vi "niRFSTS RFPM Close.vi"(11 "TSM Context":T1) -> (0 "error out":errorcluster)   [LabVIEW 2014]
uses:
  <vilib>/NI_TestStand_SemiconductorModule/NI_TestStand_Semiconductor_Module.lvlibp/PinMap/General/SemiconductorModuleContext.ctl
  <vilib>/FPGAPlugInAG/Dynamic/niLvFpga_Close_Dynamic.vi
  <vilib>/rvi/interface/nirviCloseFPGA/nirviCloseFPGA.xnode
  <vilib>/NI_TestStand_SemiconductorModule/NI_TestStand_Semiconductor_Module.lvlibp
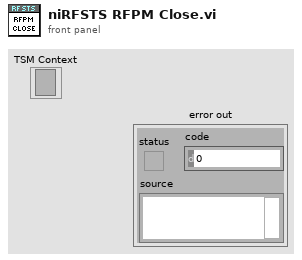
[diagram p1: front panel]
types:
  T1 = typedef "NI_TestStand_Semiconductor_Module.lvlibp/SemiconductorModuleContext.ctl" = refnum<k7>
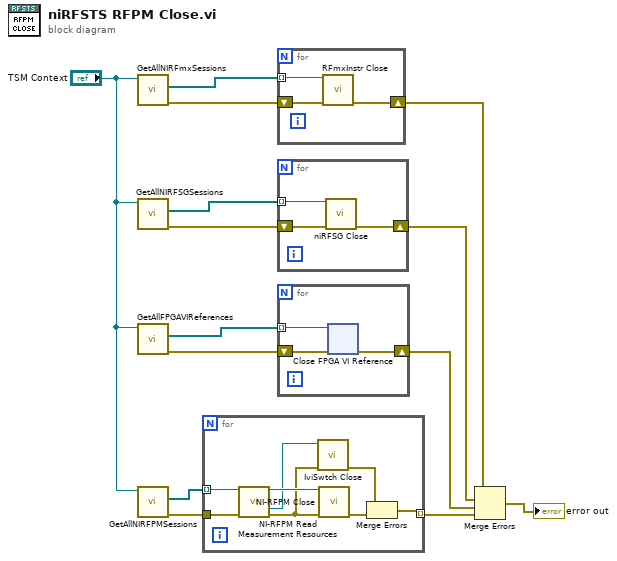
[diagram p0: block diagram]
diagram:
  n1 = call <vilib>:"GetAllNIRFmxSessions.vi"("Semiconductor Module Context"="TSM Context") -> ("error out"=w11:errorcluster, "Instrument Sessions"=w12:refnum<k21>[])  [unwired: 8 in, 1 out]
  n2 = call <vilib>:"GetAllNIRFSGSessions.vi"("Semiconductor Module Context"="TSM Context") -> ("error out"=w10:errorcluster, "Instrument Sessions"=w9:refnum<k15>[])  [unwired: 8 in, 1 out]
  n3 = call <vilib>:"GetAllFPGAVIReferences.vi"("Semiconductor Module Context"="TSM Context") -> ("error out"=w8:errorcluster, "FPGA VI References"=w7:refnum<k20>[])  [unwired: 8 in, 1 out]
  n4 = call <vilib>:"GetAllNIRFPMSessions.vi"("Semiconductor Module Context"="TSM Context") -> ("error out"=w1:errorcluster, "Instrument Sessions"=w2:refnum<k15>[])  [unwired: 8 in, 1 out]
  n5 = for {
    tunnel: w2 -> [w20] mode=indexing
    tunnel: w1 -> [w19]
    tunnel: [w22] -> w14 mode=indexing
    n6 = call <instrlib>:"NI-RFPM Read Measurement Resources.vi"("NI-5530 handle in"=w20, "error in"=w19) -> ("NI-5530 handle out"=w18:refnum<k15>, "Switch handle"=w16:refnum<k15>, "error out"=w17:errorcluster)  [unwired: 9 in, 2 out]
    n7 = call <vilib>:"IviSwtch Close.vi"("error in (no error)"=w17, "instrument handle"=w16) -> ("error out"=w15:errorcluster)  [unwired: 9 in]
    n8 = call <instrlib>:"NI-RFPM Close.vi"("NI-5530 handle in"=w18, "error in"=w17) -> ("error out"=w21:errorcluster)  [unwired: 13 in]
    n9 = Merge Errors(w15, w21) -> (w22:errorcluster)
  }
  n10 = for {
    tunnel: w12 -> [w25] mode=indexing
    shift-right: [w23] -> w6
    shift-left: w11 -> [w24]
    n11 = call <vilib>:"RFmxInstr Close.vi"("Instrument Handle In"=w25, "error in (no error)"=w24) -> ("error out"=w23:errorcluster)  [unwired: 13 in]
  }
  n12 = for {
    shift-right: [w27] -> w5
    shift-left: w10 -> [w28]
    tunnel: w9 -> [w26] mode=indexing
    n13 = call <instrlib>:"niRFSG Close.vi"("instrument handle"=w26, "error in"=w28) -> ("error out"=w27:errorcluster)  [unwired: 13 in]
  }
  n14 = for {
    shift-right: [w30] -> w4
    shift-left: w8 -> [w31]
    tunnel: w7 -> [w29] mode=indexing
    n15 = xnode "Close FPGA VI Reference"("FPGA VI Reference In"=w29, "error in"=w31) -> ("error out"=w30:errorcluster)
  }
  n16 = Merge Errors(w6, w5, w4, w14) -> (→"error out":errorcluster)
